vi "SETTING.vi"() -> ()   [LabVIEW 2017]
uses:
  <vilib>/Utility/error.llb/DialogType.ctl
  Global/Global 1.vi
panel:
  in  "COUNTER":bool
  in  "TRACEABILITY":bool
  in  "IP Setting":bool
  out "error out":errorcluster
  out "Screen Index":i32
  in  "error in (no error)":errorcluster
  in  "Home":bool
  in  "Remove":bool
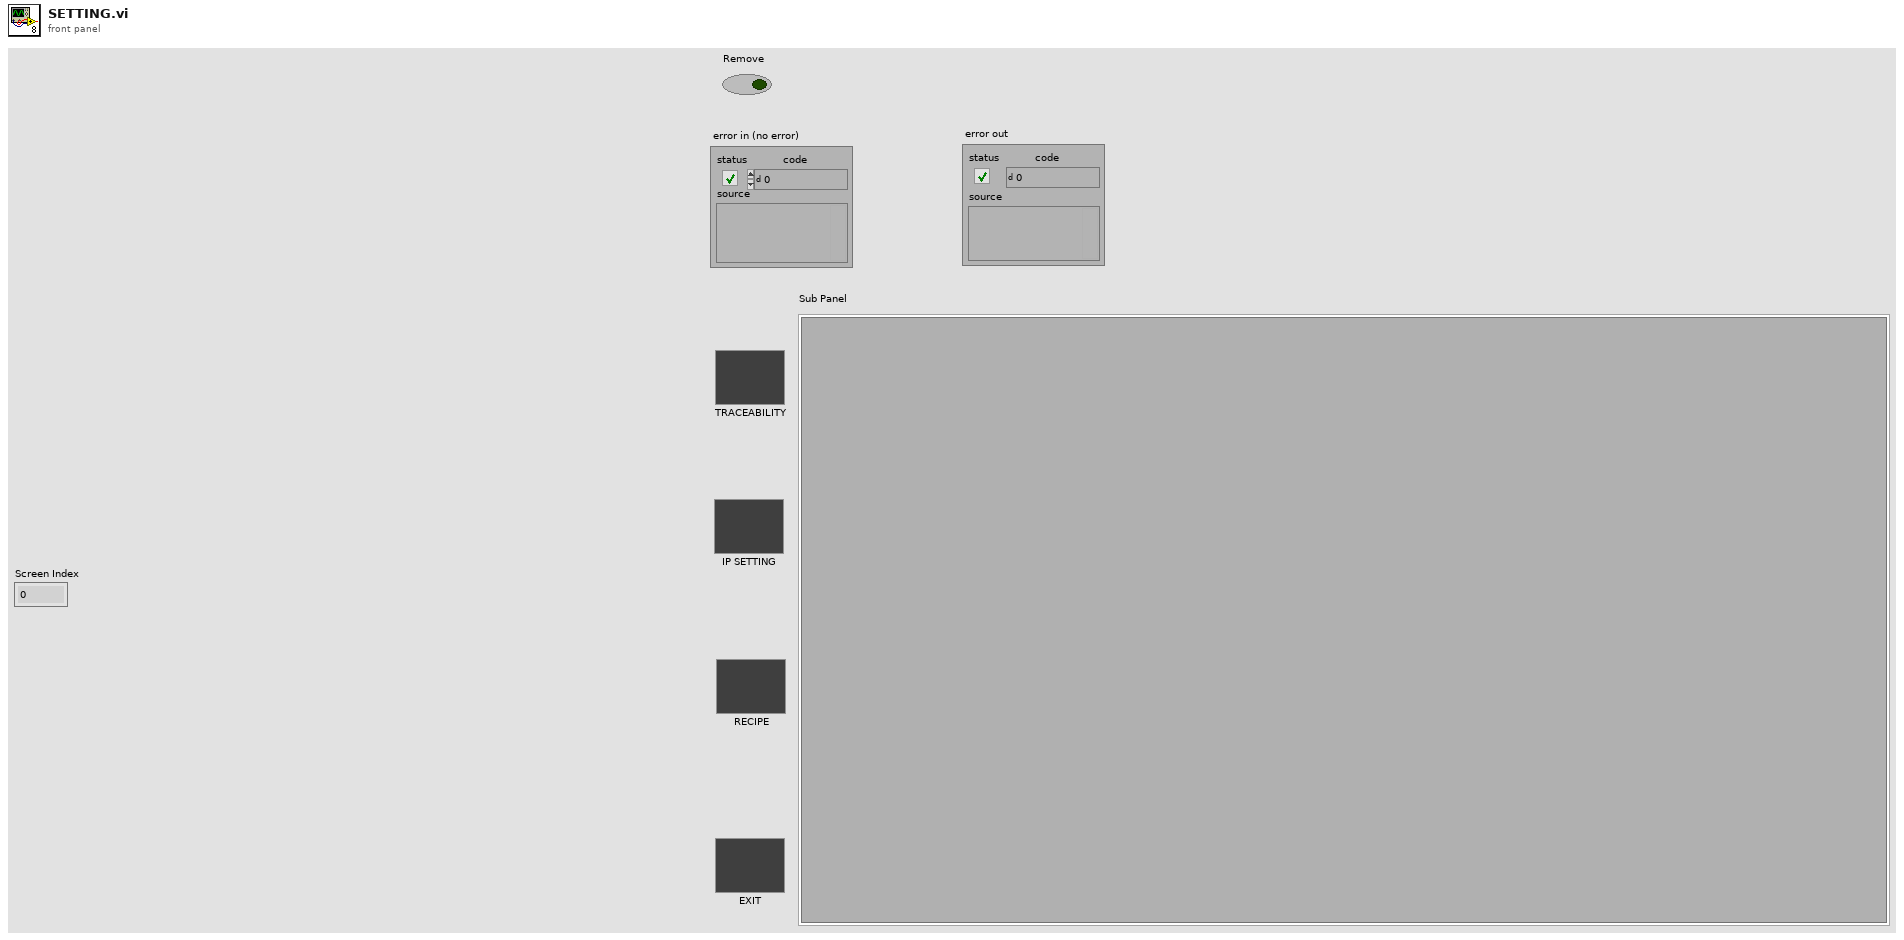
[diagram p1: front panel]
types:
  T1 = typedef "DialogType.ctl" = u16
  T2 = enum32{"invalid app kind", "Development System", "Run Time System", "Student Edition", "Embedded LabVIEW", "Evaluation", "Custom"}
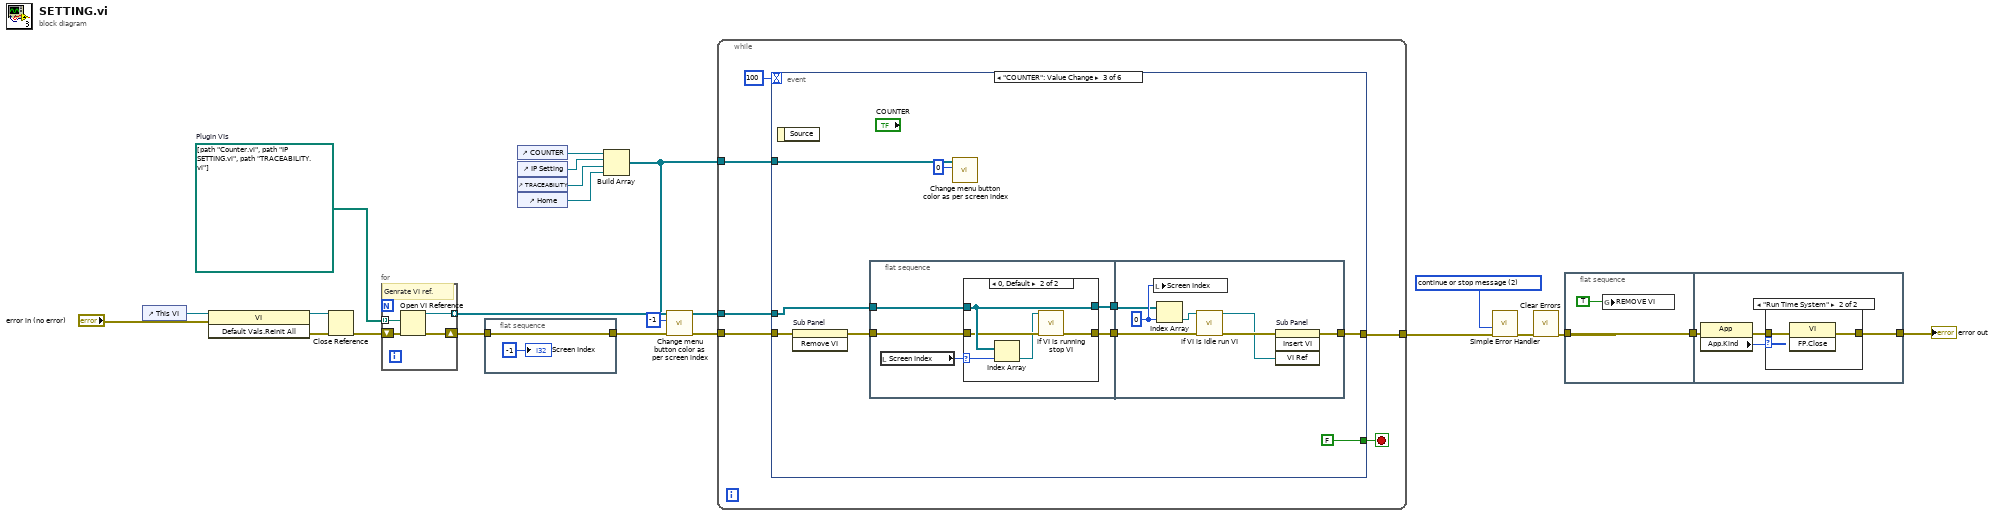
[diagram p0: block diagram]
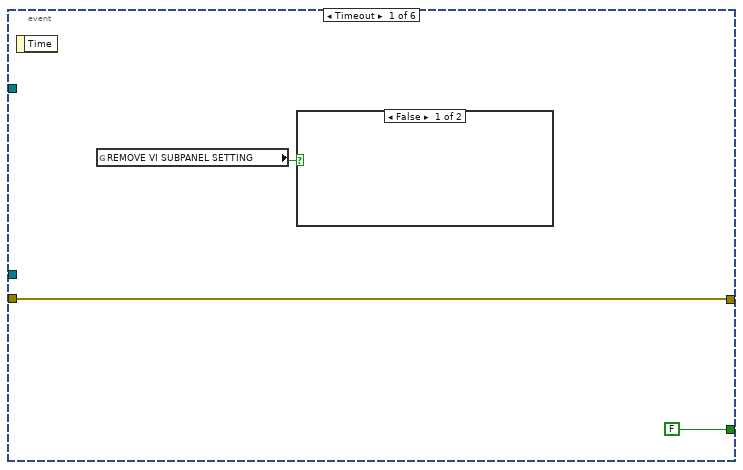
[diagram p3: hidden frame]
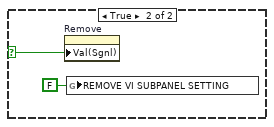
[diagram p4: hidden frame]
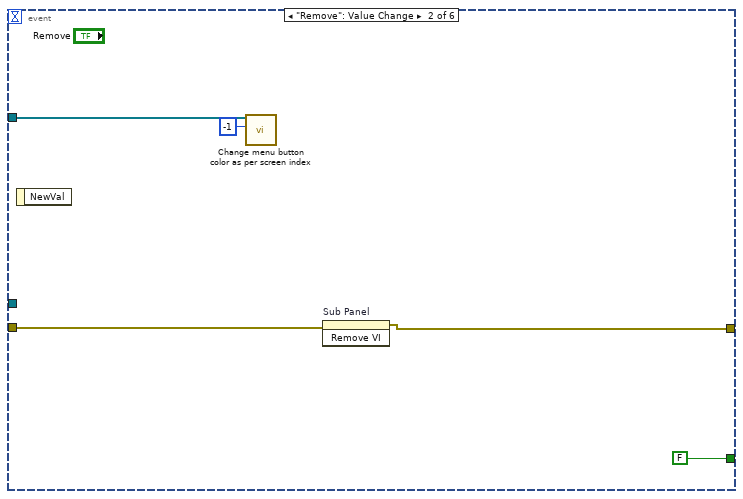
[diagram p5: hidden frame]
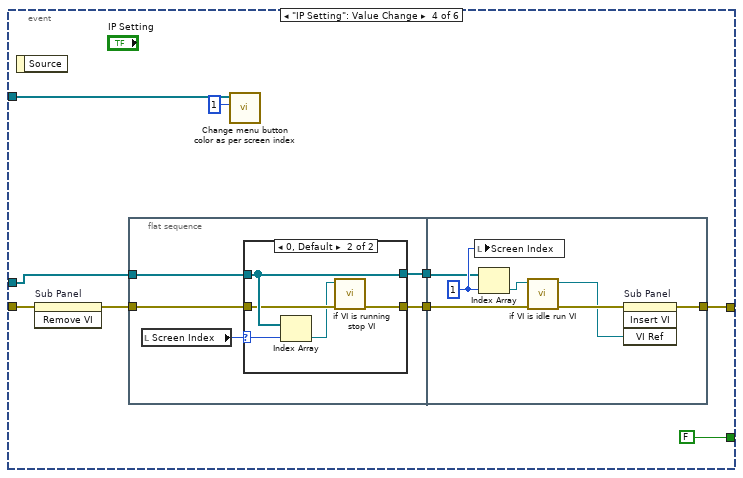
[diagram p7: hidden frame]
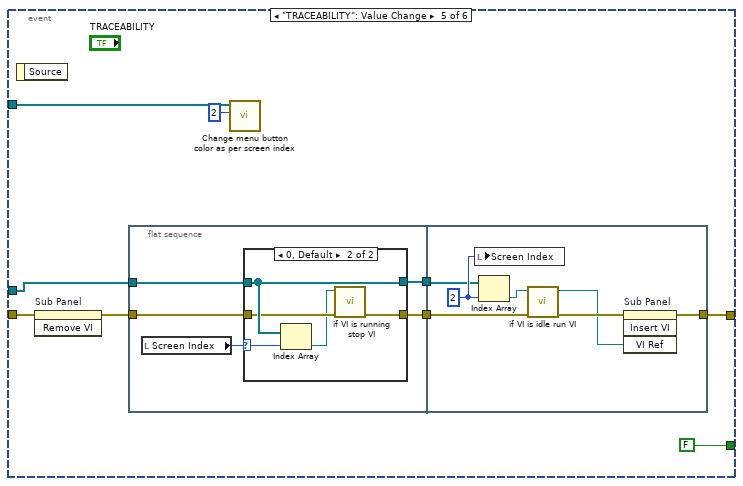
[diagram p9: hidden frame]
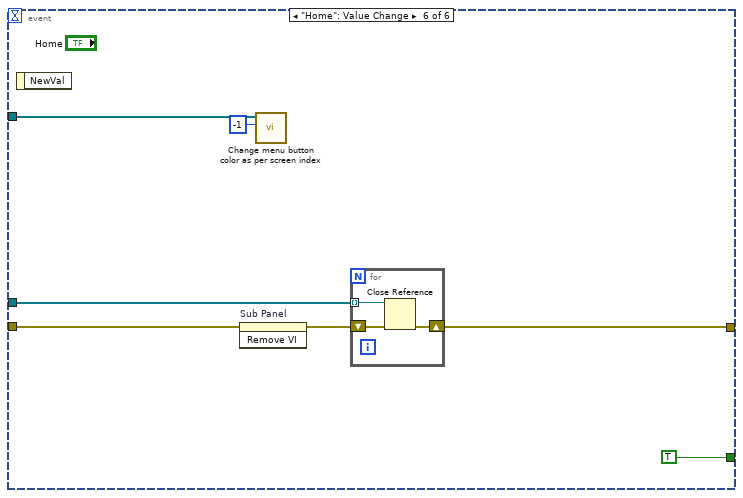
[diagram p11: hidden frame]
diagram:
  w10 = T1 2 items=["no dialog", "OK message", "continue or stop message", "OK message + warnings", "continue/stop + warnings"] ("type of dialog (OK msg:1)")
  w18 = path[] [path "Counter.vi", path "IP SETTING.vi", path "TRACEABILITY.vi"]  # Plugin VIs
  n1 = control-ref of="This VI"() -> (w21:refnum<vi>)
  n2 = invoke class="VI" method="Default Vals.Reinit All"(reference=w21, error in="error in (no error)") -> (reference out=w19:refnum<vi>, error out=w20:errorcluster)  [unwired: 1 in, 1 out]
  n3 = Close Reference(reference=w19, error in (no error)=w20) -> (error out=w17:errorcluster)
  n4 = for {
    tunnel: w18 -> [w24] mode=indexing
    tunnel: [w25] -> w14 mode=indexing
    shift-right: [w26] -> w15
    shift-left: w17 -> [w23]
    # "Genrate VI ref."
    n5 = Open VI Reference(vi path=w24, error in (no error)=w23) -> (vi reference=w25:refnum<vi>, error out=w26:errorcluster)  [unwired: 4 in]
  }
  n6 = flat-sequence {
    tunnel: w15 -> [w28]
    tunnel: [w28] -> w6
    frame #0 {
      "Screen Index" <- -1 ("Screen Index")
    }
  }
  n7 = control-ref of="COUNTER"() -> (w1:refnum<vi>)
  n8 = control-ref of="IP Setting"() -> (w4:refnum<vi>)
  n9 = control-ref of="TRACEABILITY"() -> (w3:refnum<vi>)
  n10 = control-ref of="Home"() -> (w2:refnum<vi>)
  n11 = Build Array(w1, w4, w3, w2) -> (w7:refnum<vi>[])
  n12 = call "Change menu button color as per screen index.vi"("error in (no error)"=w6, "Screen Index"=-1, "Array"=w7) -> ("error out"=w5:errorcluster)  [unwired: 8 in]
  n13 = while {
    tunnel: w5 -> [w32]
    tunnel: w14 -> [w30]
    tunnel: [w31] -> w9
    tunnel: w7 -> [w29]
    stop <- w33 stop-if-true
    n14 = event shown="[2] \"COUNTER\": Value Change" {
      selector: _ -> [_ _ _ _ _ _]
      dyn-events: _ -> [_ _ _ _ _ _]
      timeout: 100 -> [_ _ _ _ _ _]
      tunnel: [FALSE FALSE FALSE FALSE FALSE TRUE] -> w33
      tunnel: [w36 w43 w48 w76 w104 w131] -> w31
      tunnel: w32 -> [w36 w44 w50 w78 w106 w132]
      tunnel: w30 -> [_ _ w49 w77 w105 w133]
      tunnel: w29 -> [_ w40 w46 w74 w102 w130]
      event Timeout {
        n15 = event-data() -> ()  [unwired: 1 in, 1 out]
        n16 = global read "Global 1.vi" "REMOVE VI SUBPANEL SETTING"() -> (w35:bool)
        n17 = case shown="False" w35 {
          selector: w35 -> [_ w39]
          frame False {
          }
          frame True {
            n18 = property on="Remove" class="Bool (strict)"("Val(Sgnl)"=w39) -> ()  [unwired: 2 in, 2 out]
            n19 = global write "Global 1.vi" "REMOVE VI SUBPANEL SETTING"(FALSE ("REMOVE VI SUBPANEL SETTING")) -> ()
          }
        }
      }
      event "Remove": Value Change {
        n20 = event-data() -> ()  [unwired: 1 in, 1 out]
        n21 = call "Change menu button color as per screen index.vi"("Screen Index"=-1, "Array"=w40) -> ()  [unwired: 9 in, 1 out]
        n22 = invoke on="Sub Panel" class="SubPnl" method="Remove VI"(error in=w44) -> (error out=w43:errorcluster)  [unwired: 2 in, 2 out]
      }
      event "COUNTER": Value Change {
        n23 = event-data() -> ()  [unwired: 1 in, 1 out]
        n24 = invoke on="Sub Panel" class="SubPnl" method="Remove VI"(error in=w50) -> (error out=w51:errorcluster)  [unwired: 2 in, 2 out]
        n25 = flat-sequence {
          tunnel: w51 -> [w58]
          tunnel: w49 -> [w55]
          tunnel: [w57] -> w53
          tunnel: [w54] -> w52
          tunnel: [w70] -> w48
          tunnel: w53 -> [w69]
          tunnel: w52 -> [w71]
          frame #0 {
            n26 = local read "Screen Index"() -> (w56:i32)
            n27 = case shown="0, Default" w56 {
              selector: w56 -> [_ w65]
              tunnel: w58 -> [w60 w63]
              tunnel: [w60 w62] -> w57
              tunnel: w55 -> [w59 w64]
              tunnel: [w59 w64] -> w54
              frame -1 {
              }
              frame 0, Default {
                n28 = Index Array(array=w64, index=w65) -> (element=w61:refnum<vi>)
                n29 = call "if VI is running stop VI.vi"("error in (no error)"=w63, "VI in"=w61) -> ("error out"=w62:errorcluster)  [unwired: 8 in, 1 out]
              }
            }
          }
          frame #1 {
            w72 = 0 ("index")
            n30 = local write "Screen Index"(w72) -> ()
            n31 = Index Array(array=w71, index=w72) -> (element=w66:refnum<vi>)
            n32 = call "if VI is idle run VI.vi"("error in (no error)"=w69, "VI in"=w66) -> ("error out"=w68:errorcluster, "VI out"=w67:refnum<vi>)  [unwired: 8 in]
            n33 = invoke on="Sub Panel" class="SubPnl" method="Insert VI"(error in=w68, "VI Ref"=w67) -> (error out=w70:errorcluster)  [unwired: 2 in, 3 out]
          }
        }
        n34 = call "Change menu button color as per screen index.vi"("Screen Index"=0, "Array"=w46) -> ()  [unwired: 9 in, 1 out]
      }
      event "IP Setting": Value Change {
        n35 = event-data() -> ()  [unwired: 1 in, 1 out]
        n36 = invoke on="Sub Panel" class="SubPnl" method="Remove VI"(error in=w78) -> (error out=w79:errorcluster)  [unwired: 2 in, 2 out]
        n37 = flat-sequence {
          tunnel: w79 -> [w86]
          tunnel: w77 -> [w83]
          tunnel: [w85] -> w81
          tunnel: [w82] -> w80
          tunnel: [w98] -> w76
          tunnel: w81 -> [w97]
          tunnel: w80 -> [w99]
          frame #0 {
            n38 = local read "Screen Index"() -> (w84:i32)
            n39 = case shown="0, Default" w84 {
              selector: w84 -> [_ w93]
              tunnel: w86 -> [w88 w91]
              tunnel: [w88 w90] -> w85
              tunnel: w83 -> [w87 w92]
              tunnel: [w87 w92] -> w82
              frame -1 {
              }
              frame 0, Default {
                n40 = Index Array(array=w92, index=w93) -> (element=w89:refnum<vi>)
                n41 = call "if VI is running stop VI.vi"("error in (no error)"=w91, "VI in"=w89) -> ("error out"=w90:errorcluster)  [unwired: 8 in, 1 out]
              }
            }
          }
          frame #1 {
            w100 = 1 ("index")
            n42 = local write "Screen Index"(w100) -> ()
            n43 = Index Array(array=w99, index=w100) -> (element=w94:refnum<vi>)
            n44 = call "if VI is idle run VI.vi"("error in (no error)"=w97, "VI in"=w94) -> ("error out"=w96:errorcluster, "VI out"=w95:refnum<vi>)  [unwired: 8 in]
            n45 = invoke on="Sub Panel" class="SubPnl" method="Insert VI"(error in=w96, "VI Ref"=w95) -> (error out=w98:errorcluster)  [unwired: 2 in, 3 out]
          }
        }
        n46 = call "Change menu button color as per screen index.vi"("Screen Index"=1, "Array"=w74) -> ()  [unwired: 9 in, 1 out]
      }
      event "TRACEABILITY": Value Change {
        n47 = event-data() -> ()  [unwired: 1 in, 1 out]
        n48 = invoke on="Sub Panel" class="SubPnl" method="Remove VI"(error in=w106) -> (error out=w107:errorcluster)  [unwired: 2 in, 2 out]
        n49 = flat-sequence {
          tunnel: w107 -> [w114]
          tunnel: w105 -> [w111]
          tunnel: [w113] -> w109
          tunnel: [w110] -> w108
          tunnel: [w126] -> w104
          tunnel: w109 -> [w125]
          tunnel: w108 -> [w127]
          frame #0 {
            n50 = local read "Screen Index"() -> (w112:i32)
            n51 = case shown="0, Default" w112 {
              selector: w112 -> [_ w121]
              tunnel: w114 -> [w116 w119]
              tunnel: [w116 w118] -> w113
              tunnel: w111 -> [w115 w120]
              tunnel: [w115 w120] -> w110
              frame -1 {
              }
              frame 0, Default {
                n52 = Index Array(array=w120, index=w121) -> (element=w117:refnum<vi>)
                n53 = call "if VI is running stop VI.vi"("error in (no error)"=w119, "VI in"=w117) -> ("error out"=w118:errorcluster)  [unwired: 8 in, 1 out]
              }
            }
          }
          frame #1 {
            w128 = 2 ("index")
            n54 = local write "Screen Index"(w128) -> ()
            n55 = Index Array(array=w127, index=w128) -> (element=w122:refnum<vi>)
            n56 = call "if VI is idle run VI.vi"("error in (no error)"=w125, "VI in"=w122) -> ("error out"=w124:errorcluster, "VI out"=w123:refnum<vi>)  [unwired: 8 in]
            n57 = invoke on="Sub Panel" class="SubPnl" method="Insert VI"(error in=w124, "VI Ref"=w123) -> (error out=w126:errorcluster)  [unwired: 2 in, 3 out]
          }
        }
        n58 = call "Change menu button color as per screen index.vi"("Screen Index"=2, "Array"=w102) -> ()  [unwired: 9 in, 1 out]
      }
      event "Home": Value Change {
        n59 = event-data() -> ()  [unwired: 1 in, 1 out]
        n60 = invoke on="Sub Panel" class="SubPnl" method="Remove VI"(error in=w132) -> (error out=w134:errorcluster)  [unwired: 2 in, 2 out]
        n61 = call "Change menu button color as per screen index.vi"("Screen Index"=-1, "Array"=w130) -> ()  [unwired: 9 in, 1 out]
        n62 = for {
          shift-right: [w137] -> w131
          shift-left: w134 -> [w138]
          tunnel: w133 -> [w136] mode=indexing
          n63 = Close Reference(reference=w136, error in (no error)=w138) -> (error out=w137:errorcluster)
        }
      }
    }
  }
  n64 = call <vilib>:"Simple Error Handler.vi"("type of dialog (OK msg:1)"=w10, "error in (no error)"=w9) -> ("error out"=w13:errorcluster)  [unwired: 3 in, 4 out]
  n65 = call <vilib>:"Clear Errors.vi"("error in (no error)"=w13) -> ("error out"=w12:errorcluster)  [unwired: 5 in, 1 out]
  n66 = flat-sequence {
    tunnel: w12 -> [w140]
    tunnel: [w140] -> w22
    tunnel: [w141] -> w11
    tunnel: w22 -> [w142]
    frame #0 {
      n67 = global write "Global 1.vi" "REMOVE VI"(TRUE ("remove_VI")) -> ()
    }
    frame #1 {
      n68 = property class="App"(error in=w142) -> (error out=w143:errorcluster, "App.Kind"=w144:T2)  [unwired: 1 in, 1 out]
      n69 = case shown="\"Run Time System\"" w144 {
        tunnel: w143 -> [w145 w147]
        tunnel: [w145 w146] -> w141
        frame Default {
        }
        frame "Run Time System" {
          n70 = invoke class="VI" method="FP.Close"(error in=w147) -> (error out=w146:errorcluster)  [unwired: 2 in, 2 out]
        }
      }
    }
  }
  "error out" <- w11
